vi "RTmain.vi"() -> ()   [LabVIEW 2019]
uses:
  <vilib>/Platform/TimedLoop/XDataNode/timing_clust.ctl
  <vilib>/Platform/TimedLoop/XDataNode/nitl_modes.ctl
  <vilib>/Platform/TimedLoop/XDataNode/wakeup.ctl
  <vilib>/FPGAPlugInAG/cRIO-9047/niLvFpga_Open_cRIO-9047.vi
  <vilib>/rvi/interface/common/dynamic/niFpgaDynamicAddResources.vi
  <vilib>/FPGAPlugInAG/Dynamic/niLvFpga_Reset_Dynamic.vi
  <vilib>/Utility/error.llb/Error Cluster From Error Code.vi
  <vilib>/rvi/errors/niLvFpgaAdjustHostInterfaceError.vi
  <vilib>/FPGAPlugInAG/Dynamic/niLvFpga_Close_Dynamic.vi
  <vilib>/rvi/interface/nirviOpenFPGA/nirviOpenFPGA.xnode
  FPGA Bitfiles/apachedaq_FPGATarget_FPGAmain_quSq4C2-LI8.lvbitx
  FPGAmain.vi
  <vilib>/rvi/interface/nirviMethod/nirviMethod.xnode
  <vilib>/Platform/TimedLoop/XDataNode/XDataNode.xnode
  <vilib>/rvi/interface/nirviCloseFPGA/nirviCloseFPGA.xnode
  <vilib>/rvi/errors/niLvFpgaMergeErrorWithErrorCode.vi
  <vilib>/FPGAPlugInAG/Dynamic/niLvFpga_StartFifo_Dynamic.vi
  <vilib>/Platform/TimedLoop/XDataNode/XDNodeRunTimeDep.lvlib
  <vilib>/FPGAPlugInAG/Dynamic/niLvFpga_WriteFifo_Dynamic.vi
  <vilib>/FPGAPlugInAG/Dynamic/niLvFpga_ReadFifo_Dynamic.vi
panel:
  out "Log Error":errorcluster
  out "File Name":string
  out "Time":timestamp
  out "Recording":bool
  in  "Record":bool
  out "RPM":dbl
  out "RPM 2":dbl
  out "RPM 1":dbl
  out "Blk Pos (ft)":dbl
  out "Tach 2 Period (ms)":sgl
  out "Tach 1 Period (ms)":sgl
  out "Torque (ft-lbf)":sgl
  out "Torque Pin (Amp)":sgl
  out "Total Load (lbf)":sgl
  out "Load 2 (lbf)":sgl
  out "Load 1 (lbf)":sgl
  out "Load 2 (V)":sgl
  out "Load 1 (V)":sgl
  out "Blk Pos (in)":sgl
  out "Blk Pos (Amp)":sgl
  in  "Load 2 Zero":sgl
  in  "Load 1 Zero":sgl
  in  "Trq Calib Pt 1 (ft-lbf)":sgl
  in  "Trq Calib Pt 1 (Amp)":sgl
  in  "Trq Calib Pt 0 (ft-lbf)":sgl
  in  "Trq Calib Pt 0 (Amp)":sgl
  in  "Blk Calib Pt 1 (in)":sgl
  in  "Blk Calib Pt 1 (Amp)":sgl
  in  "Blk Calib Pt 0 (in)":sgl
  in  "Blk Calib Pt 0 (Amp)":sgl
  out "Stopped":bool
  out "error out":errorcluster
  in  "Stop":bool
  # "Weight-On-Bit"
  # "Rotational Speed"
  # "Torque"
  # "Block Position"
  # "Torque Calibration"
  # "Block Position Calibration"
  # "WOB Calibration"
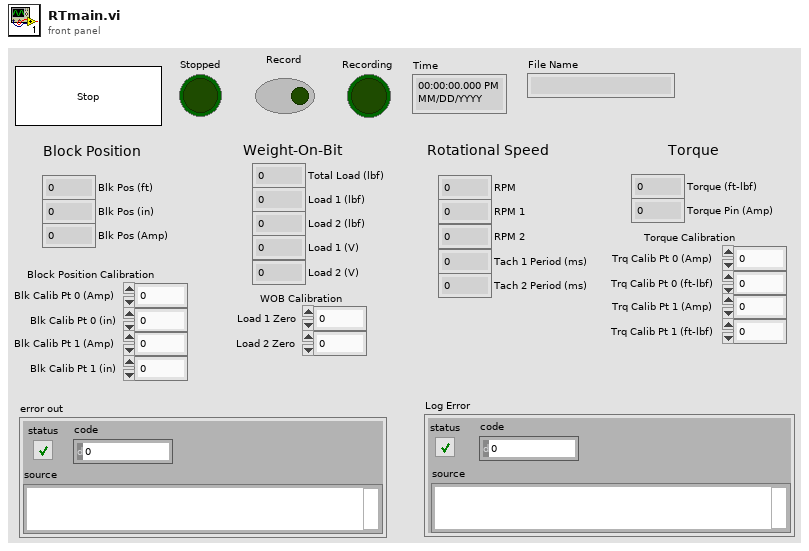
[diagram p1: front panel]
types:
  T1 = typedef "XDNodeRunTimeDep.lvlib/timing_clust.ctl" = cluster{"Expected End [f-1]":u64, "Actual End [f-1]":u64, "Finished Late? [f-1]":bool, "Expected End [i-1]":u64, "Actual End [i-1]":u64, "Finished Late? [i-1]":bool, "Expected Start [i]":u64, "Actual Start [i]":u64, "Expected Start [f]":u64, "Actual Start [f]":u64, "Source Name":string, "Structure Name":string, "Period":i64, "Deadline":i64, "Offset":i64, "Start":i64, "Priority":i32, "Timeout":i32, "Mode":T2, "Wakeup Reason":T3, "Error":errorcluster, "Source Type":string, "Secondary Source Type":string, "Global End Time":u64, "Global Start Time":u64, "Frame Duration":u64, "Iteration Duration":u64, "Assigned CPU":i32, "I/O Scan Engine Mode":u32}
  T2 = typedef "XDNodeRunTimeDep.lvlib/nitl_modes.ctl" = enum32{"No Change", "Process missed periods, maintain original phase", "Discard missed periods, maintain original phase", "Process missed periods, ignore original phase", "Discard missed periods, ignore original phase"}
  T3 = typedef "XDNodeRunTimeDep.lvlib/wakeup.ctl" = enum32{"Normal", "Aborted", "Asynchronous wakeup", "Timing source error", "Timed loop error", "Timeout"}
  T4 = enum16{"open", "open or create", "create or replace", "create", "open (read-only)"}
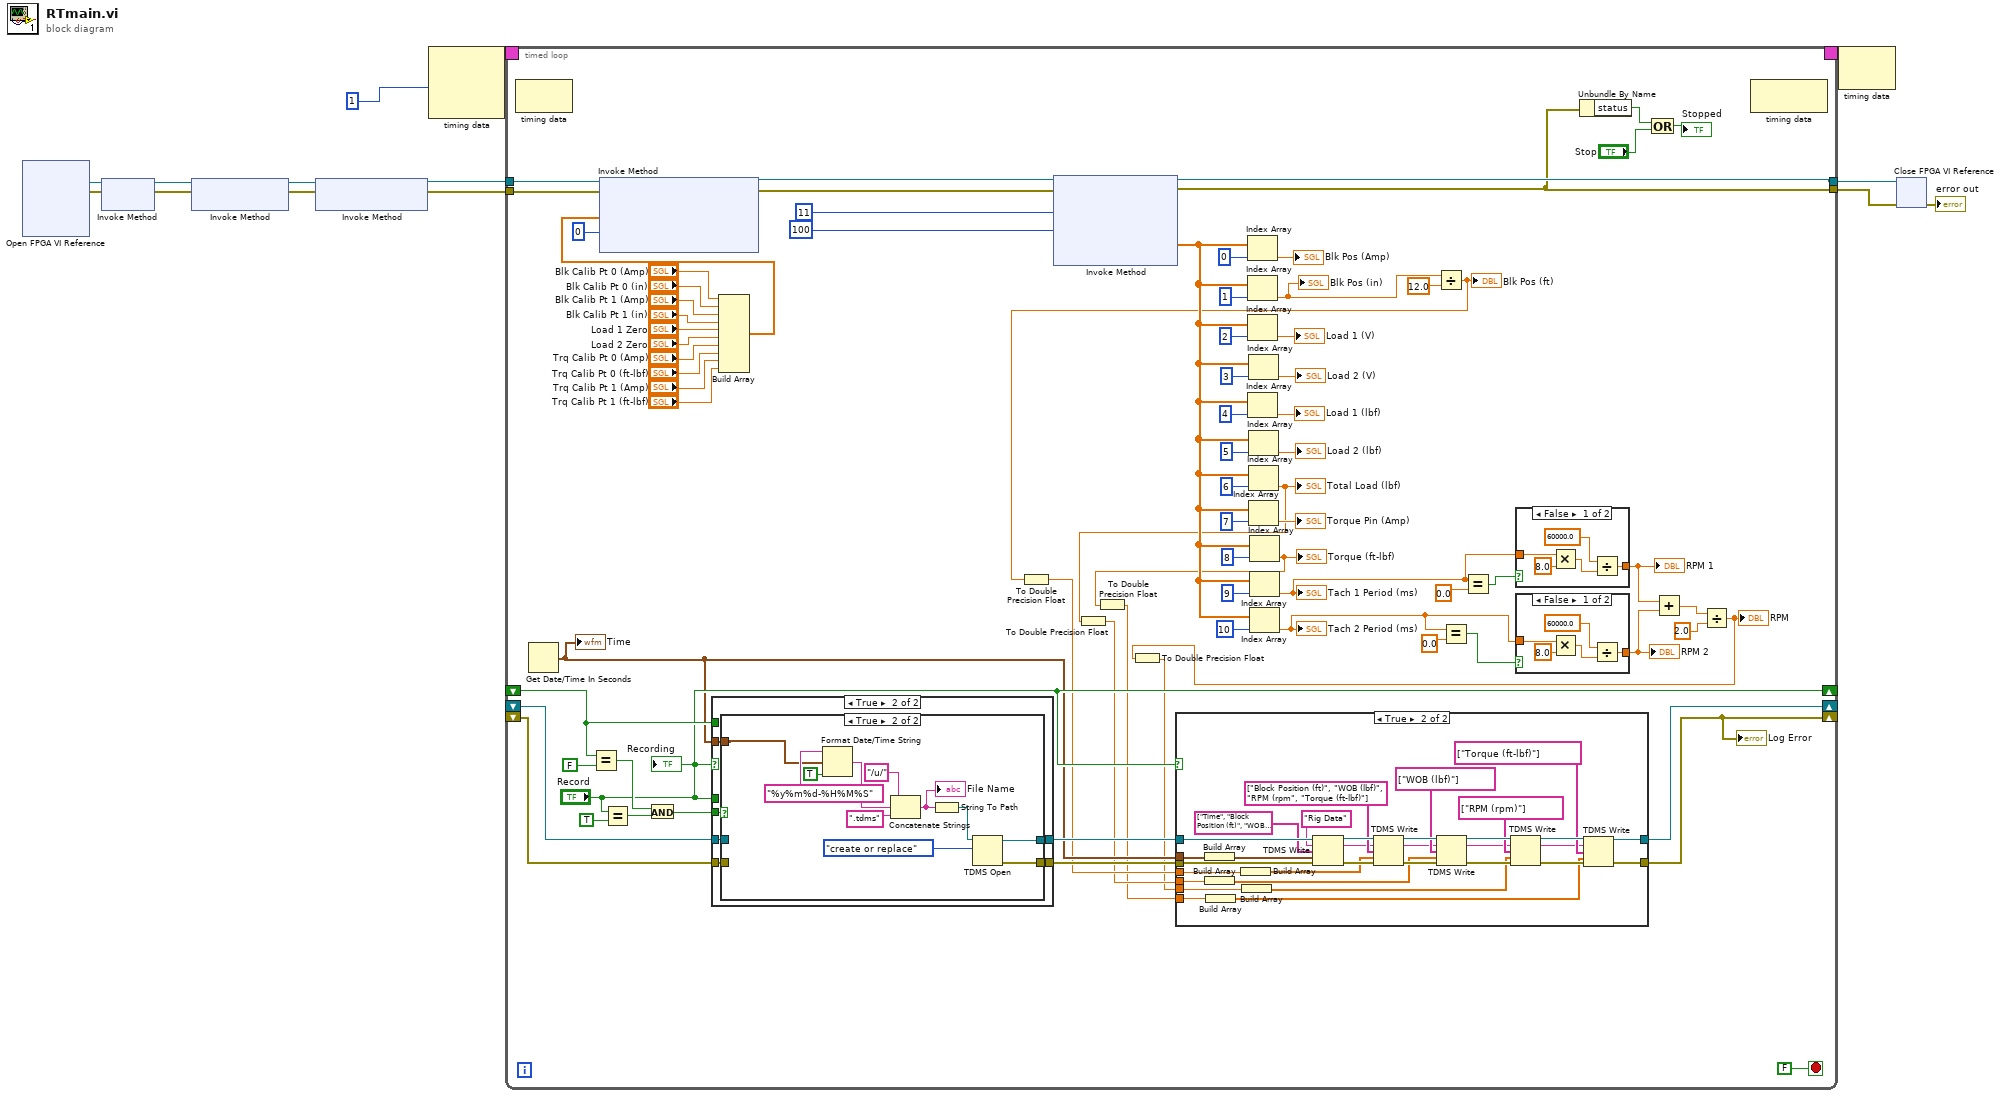
[diagram p0: block diagram]
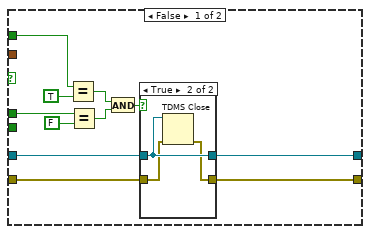
[diagram p3: hidden frame]
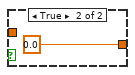
[diagram p6: hidden frame]
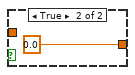
[diagram p7: hidden frame]
diagram:
  n1 = xnode "Open FPGA VI Reference"() -> ("FPGA VI Reference Out"=w9:refnum<k20>, "error out"=w8:errorcluster)  [unwired: 2 in]
  n2 = xnode "Invoke Method"("FPGA VI Reference In"=w9, "error in"=w8) -> ("FPGA VI Reference Out"=w10:refnum<k20>, "error out"=w11:errorcluster)
  n3 = xnode "Invoke Method"("FPGA VI Reference In"=w10, "error in"=w11) -> ("FPGA VI Reference Out"=w4:refnum<k20>, "error out"=w1:errorcluster)
  n4 = xnode "Invoke Method"("FPGA VI Reference In"=w4, "error in"=w1) -> ("FPGA VI Reference Out"=w3:refnum<k20>, "error out"=w2:errorcluster)
  n5 = node-c288(i64 1 ("Period")) -> (w7:T1)  [unwired: 2 in]
  n6 = timed-loop {
    tunnel: w3 -> [w87]
    tunnel: w2 -> [w86]
    tunnel: [w38] -> w14
    tunnel: [w37] -> w13
    timing: w7 -> [_]
    timing-out: [_] -> w6
    shift-right: ["Record"] -> _
    shift-left: _ -> [w31]
    shift-right: [w24] -> _
    shift-left: _ -> [w30]
    shift-right: [w26] -> _
    shift-left: _ -> [w29]
    stop <- FALSE stop-if-true
    n7 = node-c288() -> ()  [unwired: 1 in, 1 out]
    n8 = Get Date/Time In Seconds() -> (seconds since 1Jan1904=w22:timestamp)
    "Time" <- w22
    n9 = Equal?(x=w31, y=FALSE) -> (x = y?=w33:bool)
    n10 = Equal?(x="Record", y=TRUE) -> (x = y?=w34:bool)
    n11 = And(x=w33, y=w34) -> (x .and. y?=w32:bool)
    n12 = case shown="True" "Record" {
      tunnel: w32 -> [_ w146]
      tunnel: w22 -> [_ w145]
      tunnel: w31 -> [w134 _]
      tunnel: "Record" -> [w132 _]
      tunnel: [w127 w144] -> w25
      tunnel: w30 -> [w128 w143]
      tunnel: [w125 w142] -> w27
      tunnel: w29 -> [w126 w141]
      frame False {
        n13 = Equal?(x=w134, y=TRUE) -> (x = y?=w130:bool)
        n14 = Equal?(x=w132, y=FALSE) -> (x = y?=w131:bool)
        n15 = And(x=w130, y=w131) -> (x .and. y?=w129:bool)
        n16 = case shown="True" w129 {
          tunnel: w128 -> [w137 w140]
          tunnel: [w137 w140] -> w127
          tunnel: w126 -> [w136 w139]
          tunnel: [w136 w138] -> w125
          frame False {
          }
          frame True {
            n17 = TDMS Close(8:w139, 11:w140) -> (0:w138:errorcluster)  [unwired: 1 out]
          }
        }
      }
      frame True {
        n18 = case shown="True" w146 {
          tunnel: w145 -> [_ w154]
          tunnel: [w148 w153] -> w144
          tunnel: w143 -> [w148 _]
          tunnel: [w147 w152] -> w142
          tunnel: w141 -> [w147 _]
          frame False {
          }
          frame True {
            n19 = Format Date/Time String(time format string (%c)="%y%m%d-%H%M%S", seconds (now)=w154, UTC format=TRUE) -> (date/time string=w157:string)
            n20 = Concatenate Strings("/u/" ("string"), w157, ".tdms" ("string")) -> (w150:string)
            "File Name" <- w150
            n21 = String To Path(string=w150) -> (path=w149:path)
            n22 = TDMS Open(10:T4."create or replace" ("operation (0:open)"), 11:w149) -> (0:w152:errorcluster, 3:w153:refnum<k34>)  [unwired: 5 in]
          }
        }
      }
    }
    n23 = Build Array("Blk Calib Pt 0 (Amp)", "Blk Calib Pt 0 (in)", "Blk Calib Pt 1 (Amp)", "Blk Calib Pt 1 (in)", "Load 1 Zero", "Load 2 Zero", "Trq Calib Pt 0 (Amp)", "Trq Calib Pt 0 (ft-lbf)", "Trq Calib Pt 1 (Amp)", "Trq Calib Pt 1 (ft-lbf)") -> (w74:sgl[])
    n24 = xnode "Invoke Method"("FPGA VI Reference In"=w87, "error in"=w86, "Data"=w74, "Timeout (ms)"=0) -> ("FPGA VI Reference Out"=w39:refnum<k20>, "error out"=w40:errorcluster)  [unwired: 1 out]
    n25 = xnode "Invoke Method"("FPGA VI Reference In"=w39, "error in"=w40, "Number of Elements"=u32 11, "Timeout (ms)"=100) -> ("FPGA VI Reference Out"=w38:refnum<k20>, "error out"=w37:errorcluster, "Data"=w53:sgl[])  [unwired: 1 out]
    n26 = Index Array(array=w53, index=0) -> (element=→"Blk Pos (Amp)":sgl)
    n27 = Index Array(array=w53, index=1) -> (element=w49:sgl)
    "Blk Pos (in)" <- w49
    n28 = Index Array(array=w53, index=2) -> (element=→"Load 1 (V)":sgl)
    n29 = Index Array(array=w53, index=4) -> (element=→"Load 1 (lbf)":sgl)
    n30 = Index Array(array=w53, index=3) -> (element=→"Load 2 (V)":sgl)
    n31 = Index Array(array=w53, index=5) -> (element=→"Load 2 (lbf)":sgl)
    n32 = Index Array(array=w53, index=6) -> (element=w21:sgl)
    "Total Load (lbf)" <- w21
    n33 = To Double Precision Float(number=w21) -> (double precision float=w17:dbl)
    n34 = Index Array(array=w53, index=7) -> (element=→"Torque Pin (Amp)":sgl)
    n35 = Index Array(array=w53, index=8) -> (element=w19:sgl)
    "Torque (ft-lbf)" <- w19
    n36 = To Double Precision Float(number=w19) -> (double precision float=w15:dbl)
    n37 = Index Array(array=w53, index=9) -> (element=w44:sgl)
    "Tach 1 Period (ms)" <- w44
    n38 = Index Array(array=w53, index=10) -> (element=w41:sgl)
    "Tach 2 Period (ms)" <- w41
    n39 = Divide(x=w49, y=sgl 12.0) -> (x/y=w23:sgl)
    "Blk Pos (ft)" <- w23
    n40 = To Double Precision Float(number=w23) -> (double precision float=w18:dbl)
    n41 = Equal?(x=w41, y=0.0) -> (x = y?=w42:bool)
    n42 = Equal?(x=w44, y=0.0) -> (x = y?=w43:bool)
    n43 = case shown="False" w43 {
      tunnel: w44 -> [w169 _]
      tunnel: [w166 sgl 0.0] -> w46
      frame False {
        n44 = Multiply(x=w169, y=sgl 8.0) -> (x*y=w168:sgl)
        n45 = Divide(x=sgl 60000.0 ("y"), y=w168) -> (x/y=w166:sgl)
      }
      frame True {
      }
    }
    "RPM 1" <- w46
    n46 = case shown="False" w42 {
      tunnel: w41 -> [w163 _]
      tunnel: [w160 sgl 0.0] -> w45
      frame False {
        n47 = Multiply(x=w163, y=sgl 8.0) -> (x*y=w162:sgl)
        n48 = Divide(x=sgl 60000.0 ("y"), y=w162) -> (x/y=w160:sgl)
      }
      frame True {
      }
    }
    "RPM 2" <- w45
    n49 = Unbundle By Name(w37) -> ("status"=w90:bool)
    n50 = Compound Arithmetic op=OR(w90, "Stop") -> (→"Stopped":bool)
    n51 = Add(x=w46, y=w45) -> (x+y=w48:sgl)
    n52 = Divide(x=w48, y=sgl 2.0) -> (x/y=w20:sgl)
    "RPM" <- w20
    n53 = To Double Precision Float(number=w20) -> (double precision float=w16:dbl)
    n54 = case shown="True" "Record" {
      tunnel: w27 -> [w92 w124]
      tunnel: [w92 w113] -> w26
      tunnel: w25 -> [w91 w123]
      tunnel: [w91 w109] -> w24
      tunnel: w18 -> [_ w105]
      tunnel: w22 -> [_ w118]
      tunnel: w17 -> [_ w102]
      tunnel: w16 -> [_ w101]
      tunnel: w15 -> [_ w99]
      frame False {
      }
      frame True {
        n55 = Build Array(w118) -> (w117:timestamp[])
        n56 = Build Array(w102) -> (w103:dbl[])
        n57 = Build Array(w99) -> (w98:dbl[])
        n58 = Build Array(w105) -> (w104:dbl[])
        n59 = Build Array(w101) -> (w100:dbl[])
        n60 = TDMS Write(0:w123, 5:"Rig Data" ("group name in (Untitled)"), 7:string[] ["Time", "Block Position (ft)", "WOB (lbf)", "RPM (rpm)", "Torque (ft-lbf)"] ("channel name(s) in (Untitled)"), 9:w117, 11:w124) -> (4:w121:refnum<k34>, 6:w96:string, 15:w120:errorcluster)  [unwired: 1 in, 1 out]
        n61 = TDMS Write(0:w121, 5:w96, 7:string[] ["Block Position (ft)", "WOB (lbf)", "RPM (rpm", "Torque (ft-lbf)"] ("channel name(s) in (Untitled)"), 9:w104, 11:w120) -> (4:w112:refnum<k34>, 6:w95:string, 15:w116:errorcluster)  [unwired: 1 in, 1 out]
        n62 = TDMS Write(0:w112, 5:w95, 7:string[] ["WOB (lbf)"] ("channel name(s) in (Untitled)"), 9:w103, 11:w116) -> (4:w111:refnum<k34>, 6:w94:string, 15:w115:errorcluster)  [unwired: 1 in, 1 out]
        n63 = TDMS Write(0:w111, 5:w94, 7:string[] ["RPM (rpm)"] ("channel name(s) in (Untitled)"), 9:w100, 11:w115) -> (4:w110:refnum<k34>, 6:w93:string, 15:w114:errorcluster)  [unwired: 1 in, 1 out]
        n64 = TDMS Write(0:w110, 5:w93, 7:string[] ["Torque (ft-lbf)"] ("channel name(s) in (Untitled)"), 9:w98, 11:w114) -> (4:w109:refnum<k34>, 15:w113:errorcluster)  [unwired: 1 in, 2 out]
      }
    }
    "Log Error" <- w26
    n65 = node-c288() -> ()  [unwired: 1 in, 1 out]
    "Recording" <- "Record"
  }
  n66 = node-c288(w6) -> ()  [unwired: 1 out]
  n67 = xnode "Close FPGA VI Reference"("FPGA VI Reference In"=w14, "error in"=w13) -> ("error out"=→"error out":errorcluster)
